vi "Start Storage Wrapper.vi"(8 "error in (no error)":errorcluster, 10 "Key Expression":string, 11 "Session in":u64) -> (0 "error out":errorcluster, 2 "Storage Handle":u64)   [LabVIEW 2021, in "Zenoh.lvclass"]
doc: "In Zenoh, the key expression (KE) used when creating an in-memory storage acts as the subscription pattern and addressing boundary for that storage. It defines which data, published on the network, the storage will automatically subscribe to, retain, and serve in response to queries. Essentially, the key expression acts as the filter for ingestion (what to store) and the identifier for retrieval (what to query). \n\nHere are the specific uses of the key expression in this context:\n\n- Definition of Scope (Subscription): It determines the set of keys the storage will store. Using wildcards (* for a single chunk, ** for any number of chunks) allows a single storage instance to capture a wide range of hierarchical data (e.g., robot/sensor/** to store all sensor data from all robots).\n\n- Queryable Addressing: The storage acts as a queryable, and this key expression determines which get requests (queries) it will respond to. If a query matches the storage's key expression, the storage returns the stored data.\n\n- Data Organization: It helps organize the internal storage structure, allowing the system to efficiently store and retrieve data based on hierarchical paths.\n\n- Replication/Alignment: In scenarios with multiple storages, the key expression is used by the anti-entropy protocol to ensure that storages subscribed to the same (or overlapping) key expressions remain consistent, enabling data synchronization."
uses:
  Zenoh.lvclass
  Zenoh.lvclass/Zenoh.ctl
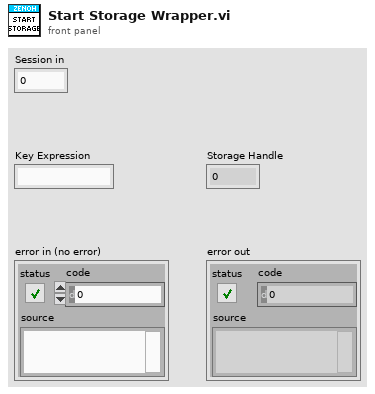
[diagram p1: front panel]
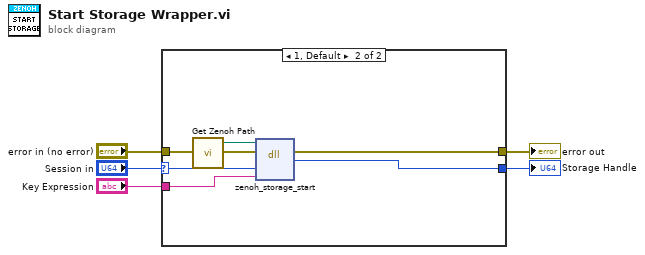
[diagram p0: block diagram]
diagram:
  n1 = case shown="1, Default" "Session in" {
    selector: "Session in" -> [_ w10]
    tunnel: [w6 w8] -> w5
    tunnel: "error in (no error)" -> [w6 w11]
    tunnel: [_ w9] -> w3
    tunnel: "Key Expression" -> [_ w7]
    frame 0 {
    }
    frame 1, Default {
      n2 = call "Get Zenoh Path.vi"() -> ("Library Path"=w12:path)  [unwired: 4 in]
      n3 = dll-call lib="C:/Program Files/CIF_Foundation/Libraries/zenoh_lv_wrapper.dll" fn="zenoh_storage_start"(path in=w12, error in=w11, "session_prt"=w10, "key_expr"=w7) -> (error out=w8:errorcluster, "LivelinessToken"=w9:u64)  [unwired: 3 in, 1 out]
    }
  }
  "error out" <- w5
  "Storage Handle" <- w3
